vi "Process-message.vi"(8 "error in (no error)":errorcluster, 10 "Message":refnum<class "Message.lvclass">, 11 "ModComm in":T1) -> (0 "error out":errorcluster, 1 "Exit?":bool, 3 "ModComm out":T1)   [LabVIEW 2013, in "Server.lvlib" / "Server.lvclass"]
uses:
  Server.lvclass
  Object-reference.ctl
  Messages/Sources/Message.lvclass
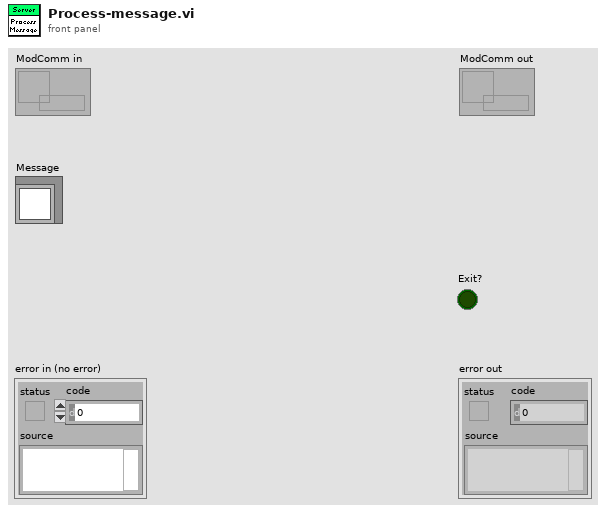
[diagram p1: front panel]
types:
  T1 = typedef "Server.lvlib/Server.lvclass/Object-reference.ctl" = refnum<data-value>
  T2 = typedef "Server.lvlib/Server.lvclass/Server-messages.ctl" = enum16{"Heartbeat", "Error", "Start client", "Client stopped", "Query status", "Send status", "Get clients"}
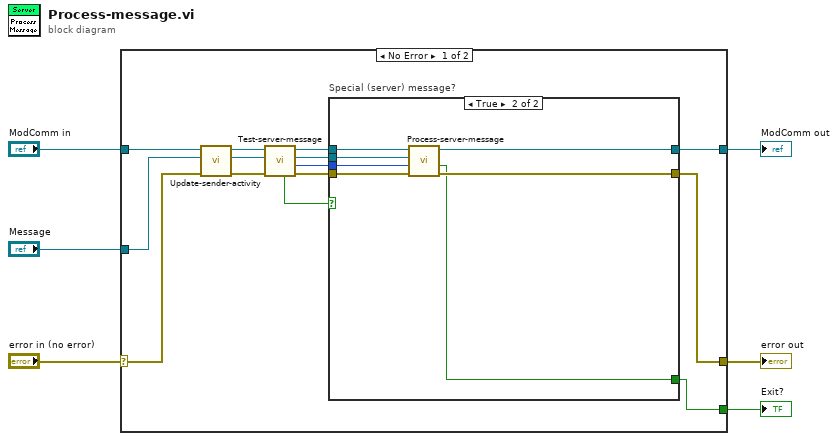
[diagram p0: block diagram]
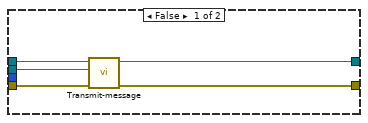
[diagram p2: hidden frame]
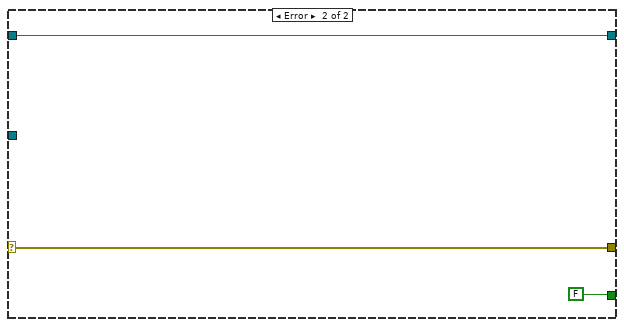
[diagram p3: hidden frame]
diagram:
  n1 = case shown="No Error" "error in (no error)" {
    selector: "error in (no error)" -> [w8 w35]
    tunnel: [w16 w35] -> w5
    tunnel: [w17 w34] -> w3
    tunnel: "ModComm in" -> [w12 w34]
    tunnel: [w15 FALSE] -> w2
    tunnel: "Message" -> [w7 _]
    frame No Error {
      n2 = call "Update-sender-activity.vi"("error in (no error)"=w8, "Message"=w7, "ModComm in"=w12) -> ("error out"=w9:errorcluster, "Message dup"=w10:refnum<class "Message.lvclass">, "ModComm out"=w11:T1)  [unwired: 6 in]
      n3 = call "Test-server-message.vi"("error in (no error)"=w9, "Message"=w10, "ModComm in"=w11) -> ("error out"=w18:errorcluster, "Server message type"=w13:T2, "Message dup"=w19:refnum<class "Message.lvclass">, "ModComm out"=w20:T1, "Server message?"=w14:bool)  [unwired: 4 in]
      n4 = case "Special (server) message?" shown="True" w14 {
        tunnel: w20 -> [w25 w31]
        tunnel: w19 -> [w23 w32]
        tunnel: w18 -> [w24 w29]
        tunnel: [w22 w28] -> w16
        tunnel: [w21 w30] -> w17
        tunnel: [_ w27] -> w15
        tunnel: w13 -> [_ w26]
        frame False {
          n5 = call "Transmit-message.vi"("error in (no error)"=w24, "Message"=w23, "ModComm in"=w25) -> ("error out"=w22:errorcluster, "ModComm out"=w21:T1)  [unwired: 7 in]
        }
        frame True {
          n6 = call "Process-server-message.vi"("error in (no error)"=w29, "Message type"=w26, "Message"=w32, "ModComm in"=w31) -> ("error out"=w28:errorcluster, "Exit?"=w27:bool, "ModComm out"=w30:T1)  [unwired: 5 in]
        }
      }
    }
    frame Error {
    }
  }
  "error out" <- w5
  "ModComm out" <- w3
  "Exit?" <- w2
